vi "b1.vi"() -> ()   [LabVIEW 2015]
panel:
  out "b":bool
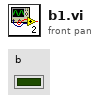
[diagram p1: front panel]
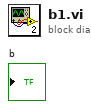
[diagram p0: block diagram]
diagram:
